vi "CreateGraphMenu_OnCurve.vi"(4 "isFloatXY":T1, 6 "isShowYvalue":T1, 9 "Language":refnum<vi>, 11 "菜单输入":refnum<k9>) -> ()   [LabVIEW 2015]
uses:
  Ctrls/YesOrNo.ctl
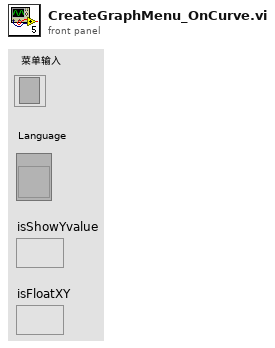
[diagram p1: front panel]
types:
  T1 = typedef "YesOrNo.ctl" = bool
  T2 = cluster{"MenuNames":string[], "MenuTags":string[]}
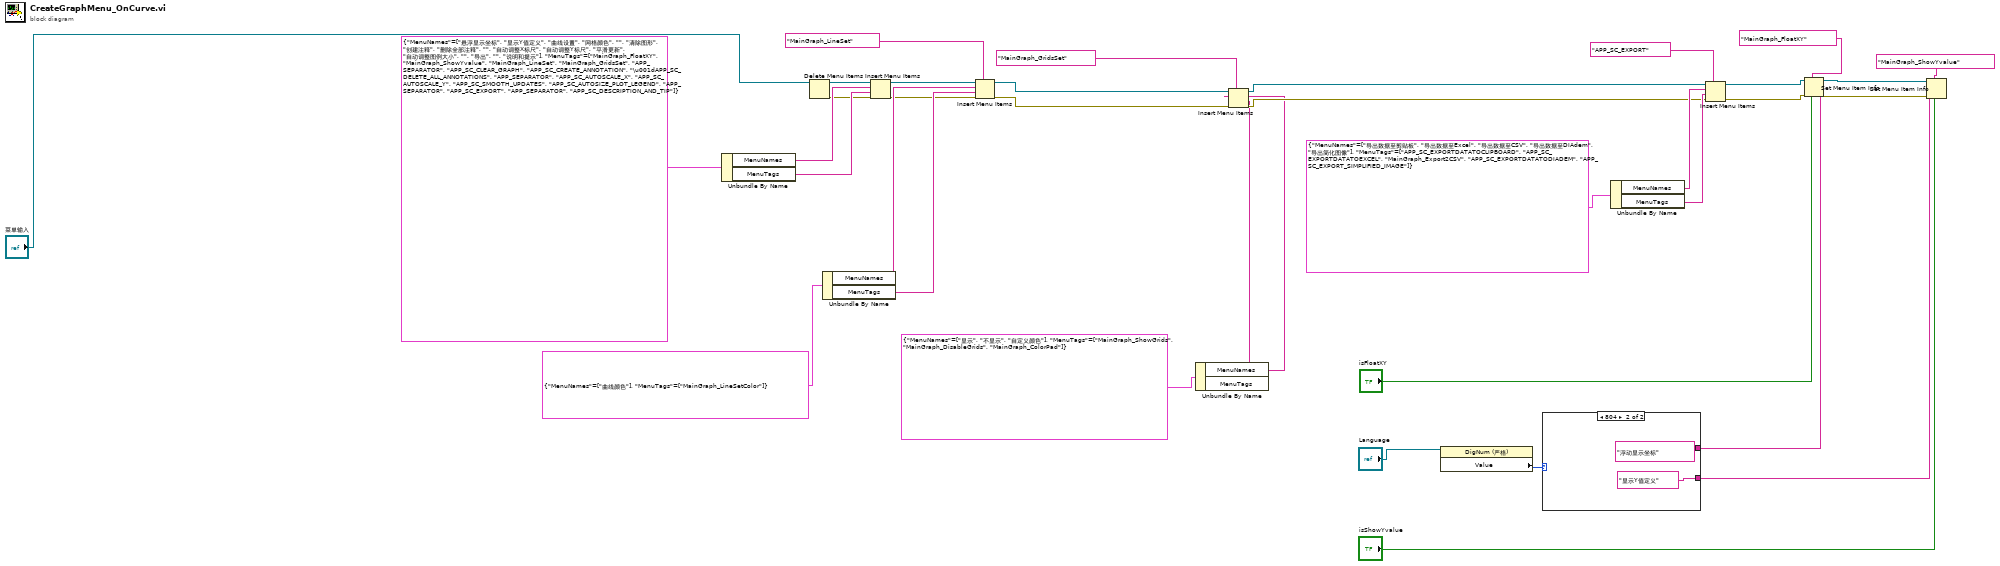
[diagram p0: block diagram]
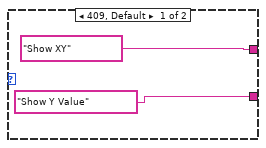
[diagram p2: hidden frame]
diagram:
  n1 = Unbundle By Name(T2 {"MenuNames"=["悬浮显示坐标", "显示Y值定义", "曲线设置", "网格颜色", "", "清除图形", "创建注释", "删除全部注释", "", "自动调整X标尺", "自动调整Y标尺", "平滑更新", "自动调整图例大小", "", "导出", "", "说明和提示"], "MenuTags"=["MainGraph_FloatXY", "MainGraph_ShowYvalue", "MainGraph_LineSet", "MainGraph_GridsSet", "APP_SEPARATOR", "APP_SC_CLEAR_GRAPH", "APP_SC_CREATE_ANNOTATION", "\u001dAPP_SC_DELETE_ALL_ANNOTATIONS", "APP_SEPARATOR", "APP_SC_AUTOSCALE_X", "APP_SC_AUTOSCALE_Y", "APP_SC_SMOOTH_UPDATES", "APP_SC_AUTOSIZE_PLOT_LEGEND", "APP_SEPARATOR", "APP_SC_EXPORT", "APP_SEPARATOR", "APP_SC_DESCRIPTION_AND_TIP"]}) -> ("MenuNames"=w22:string[], "MenuTags"=w23:string[])
  n2 = Delete Menu Items(9:"菜单输入") -> (0:w13:errorcluster, 3:w16:refnum<k9>)  [unwired: 3 in]
  n3 = Unbundle By Name(T2 {"MenuNames"=["曲线颜色"], "MenuTags"=["MainGraph_LineSetColor"]}) -> ("MenuNames"=w26:string[], "MenuTags"=w25:string[])
  n4 = Insert Menu Items(6:w13, 7:w23, 8:w22, 9:w16) -> (0:w15:errorcluster, 3:w20:refnum<k9>)  [unwired: 2 in, 1 out]
  n5 = Insert Menu Items(5:"MainGraph_LineSet" ("L10n_menu tag"), 6:w15, 7:w25, 8:w26, 9:w20) -> (0:w14:errorcluster, 3:w19:refnum<k9>)  [unwired: 1 in, 1 out]
  n6 = Unbundle By Name(T2 {"MenuNames"=["显示", "不显示", "自定义颜色"], "MenuTags"=["MainGraph_ShowGrids", "MainGraph_DisableGrids", "MainGraph_ColorPad"]}) -> ("MenuNames"=w28:string[], "MenuTags"=w29:string[])
  n7 = Insert Menu Items(5:"MainGraph_GridsSet" ("L10n_menu tag"), 6:w14, 7:w29, 8:w28, 9:w19) -> (0:w31:errorcluster, 3:w32:refnum<k9>)  [unwired: 1 in, 1 out]
  n8 = property class="DigNum (严格)"(reference="Language") -> ("Value"=w5:u32)  [unwired: 1 in, 2 out]
  n9 = case shown="804" w5 {
    tunnel: ["Show XY" "浮动显示坐标"] -> w9
    tunnel: ["Show Y Value" "显示Y值定义"] -> w10
    frame 409, Default {
    }
    frame 804 {
    }
  }
  n10 = Unbundle By Name(T2 {"MenuNames"=["导出数据至剪贴板", "导出数据至Excel", "导出数据至CSV", "导出数据至DIAdem", "导出简化图像"], "MenuTags"=["APP_SC_EXPORTDATATOCLIPBOARD", "APP_SC_EXPORTDATATOEXCEL", "MainGraph_Export2CSV", "APP_SC_EXPORTDATATODIADEM", "APP_SC_EXPORT_SIMPLIFIED_IMAGE"]}) -> ("MenuNames"=w34:string[], "MenuTags"=w35:string[])
  n11 = Insert Menu Items(5:"APP_SC_EXPORT" ("L10n_menu tag"), 6:w31, 7:w35, 8:w34, 9:w32) -> (0:w3:errorcluster, 3:w4:refnum<k9>)  [unwired: 1 in, 1 out]
  n12 = Set Menu Item Info(6:"isFloatXY", 7:"MainGraph_FloatXY", 8:w3, 10:w9, 11:w4) -> (0:w2:errorcluster)  [unwired: 2 in, 1 out]
  n13 = Set Menu Item Info(6:"isShowYvalue", 7:"MainGraph_ShowYvalue", 8:w2, 10:w10, 11:w4) -> ()  [unwired: 2 in, 2 out]
